vi "Mode Page.vi"(8 "Error in":errorcluster, 11 "INL DNL Test in":refnum<class "INL DNL Test.lvclass">=refnum) -> (0 "Error out":errorcluster, 3 "INL DNL Test out":refnum<class "INL DNL Test.lvclass">)   [LabVIEW 2020, in "INL DNL Test.lvclass"]
doc: "Mode page to select the device mode and enter the device values."
uses:
  INL DNL Test.lvclass
  D:/SDLC/Class/INL DNL Test/Test/Parent/Test.lvclass
  Class/INL DNL Test/Device/Children/Children/ADC/ADC.lvclass
  Class/INL DNL Test/Device/Children/Children/DAC/DAC.lvclass
  Typedef/User event controls.ctl
  Typedef/Queue Operation.ctl
  Class/INL DNL Test/Device/Parent/Device.lvclass
  INL DNL Test.lvclass/INL DNL Test.ctl
  DNL INL Test.lvlib
panel:
  in  "Error Rate (in %)":dbl=25.0 min=0.0 max=100.0
  in  "Voltage (V)":dbl=8.0 min=0.0
  in  "Resolution":dbl=3.0 min=1.0
  in  "DAC":bool caption="Digital to Analog converter"
  in  "ADC":bool caption="Analog to digital converter"
  # "Note:\n1. Choose the mode to calculate INL and DNl result\n2. Enter the parameter values for the calculation"
  # "Choose the mode"
  # "Enter parameters"
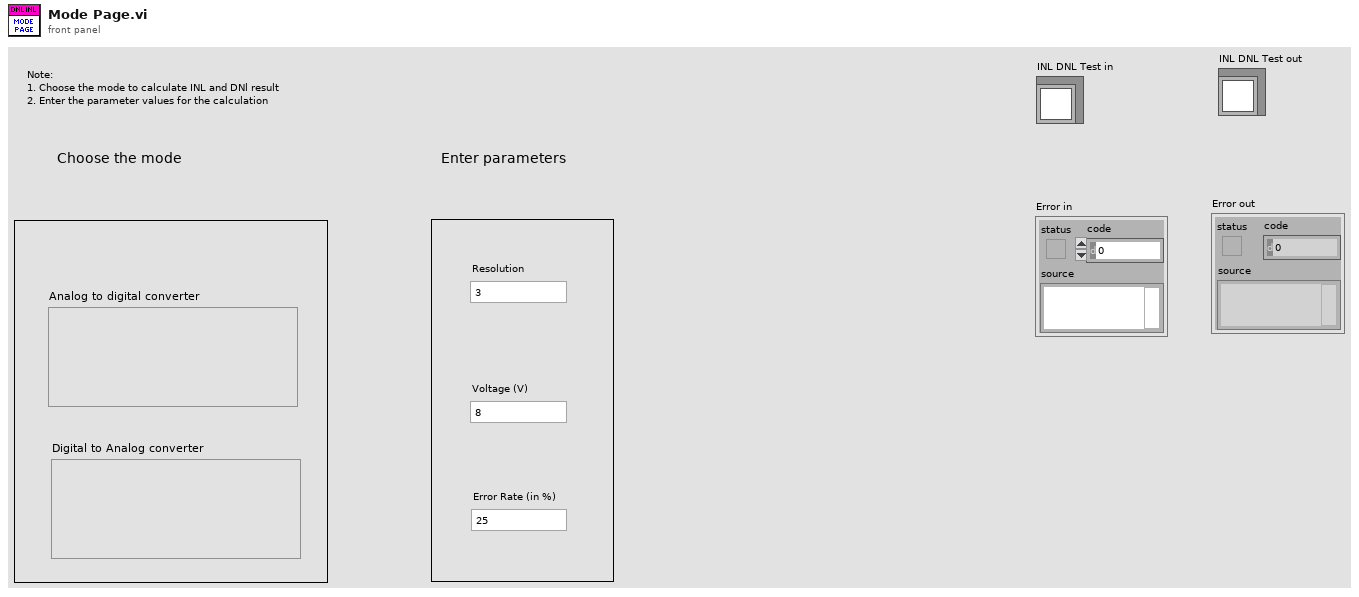
[diagram p1: front panel]
types:
  T1 = typedef "DNL INL Test.lvlib/Queue Operation.ctl" = enum16{"Create Queue", "Enqueue", "Dequeue", "Enstack", "Flush Queue", "Release Queue"}
  T2 = typedef "DNL INL Test.lvlib/User event controls.ctl" = enum16{"Create", "Generate", "Run Test", "Get Ref", "Destroy"}
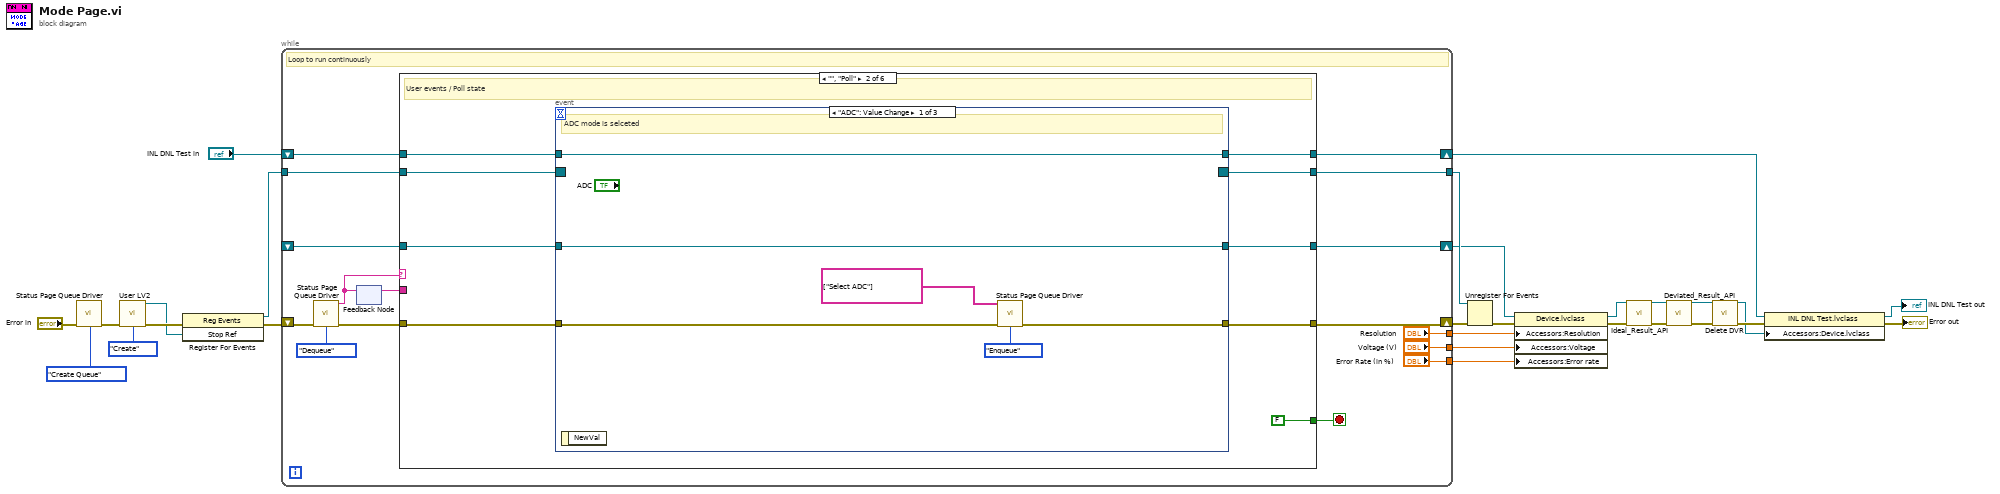
[diagram p0: block diagram]
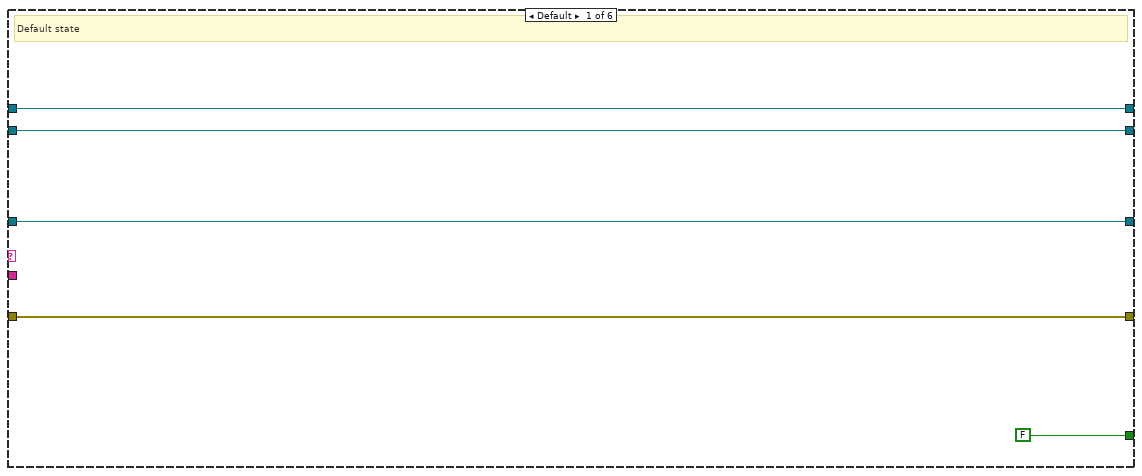
[diagram p2: hidden frame]
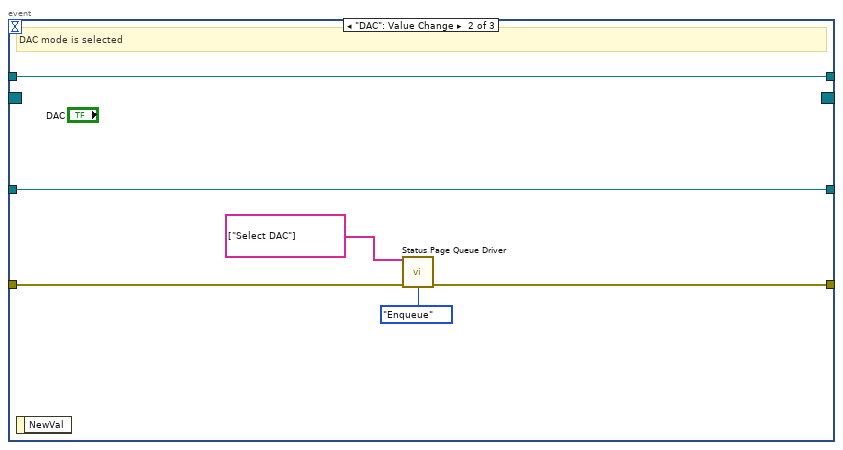
[diagram p3: hidden frame]
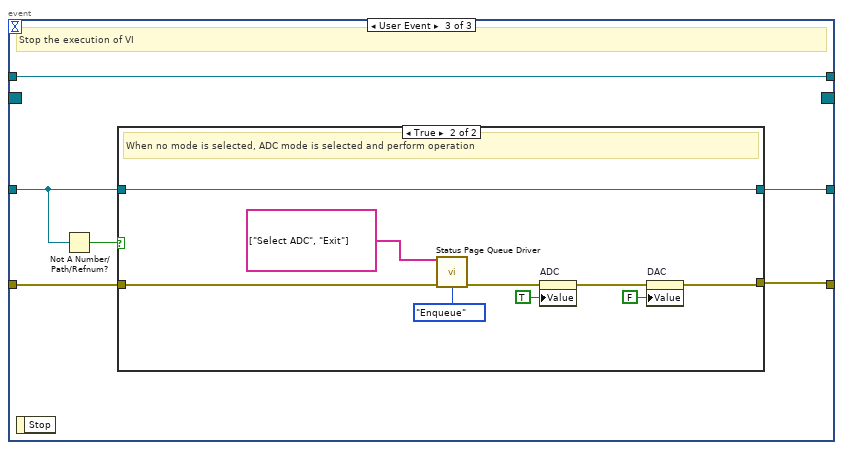
[diagram p4: hidden frame]
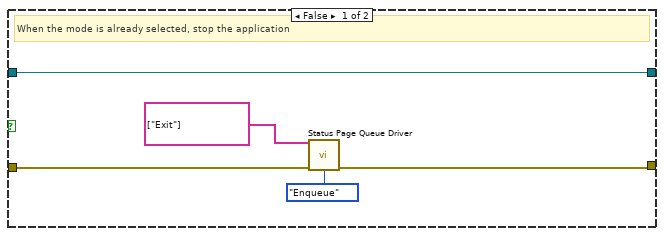
[diagram p5: hidden frame]
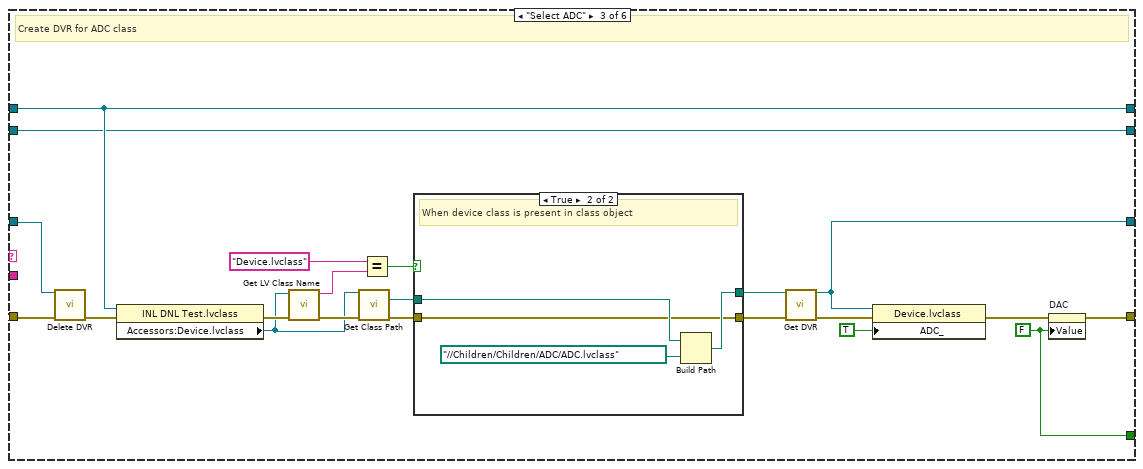
[diagram p6: hidden frame]
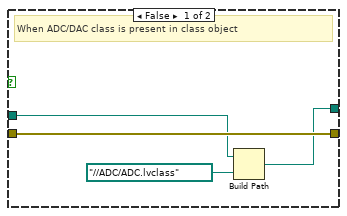
[diagram p7: hidden frame]
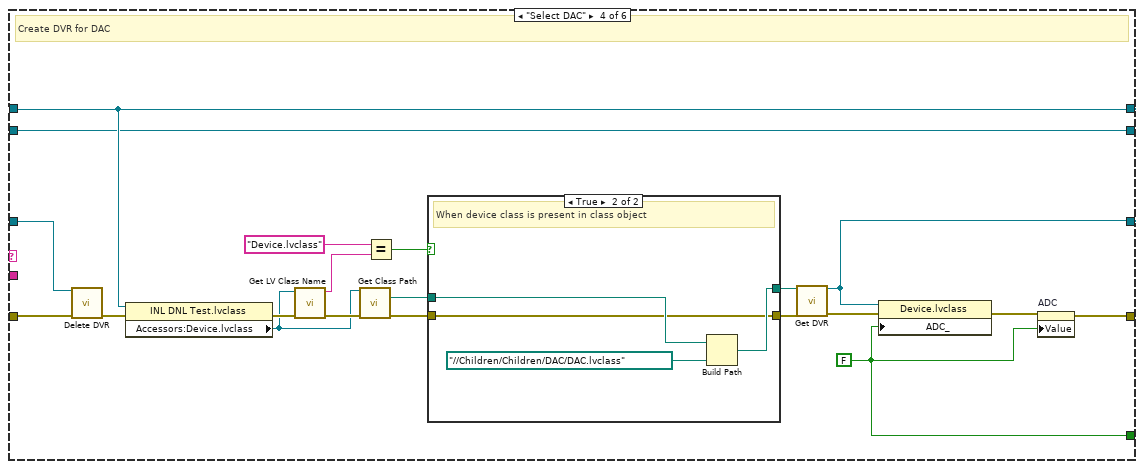
[diagram p8: hidden frame]
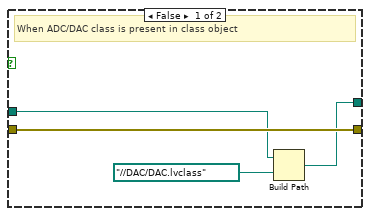
[diagram p9: hidden frame]
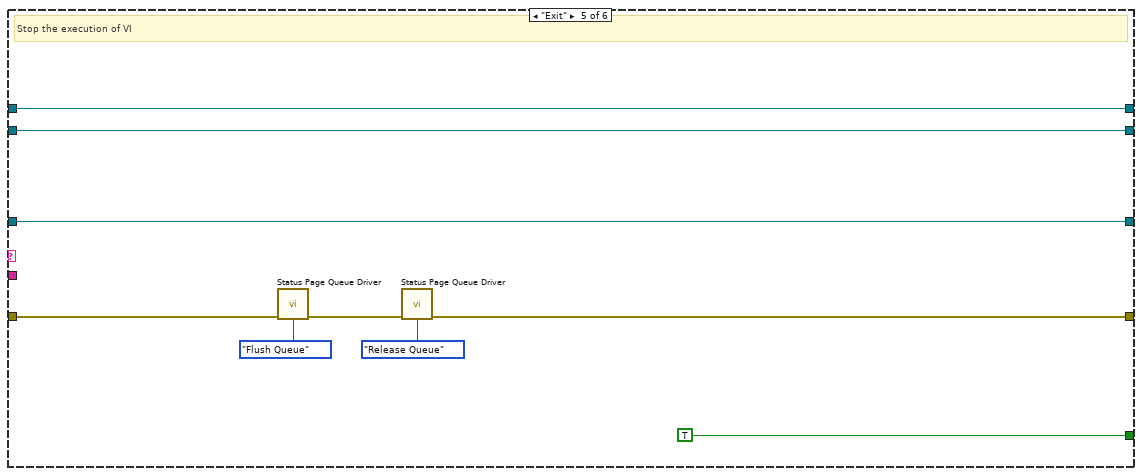
[diagram p10: hidden frame]
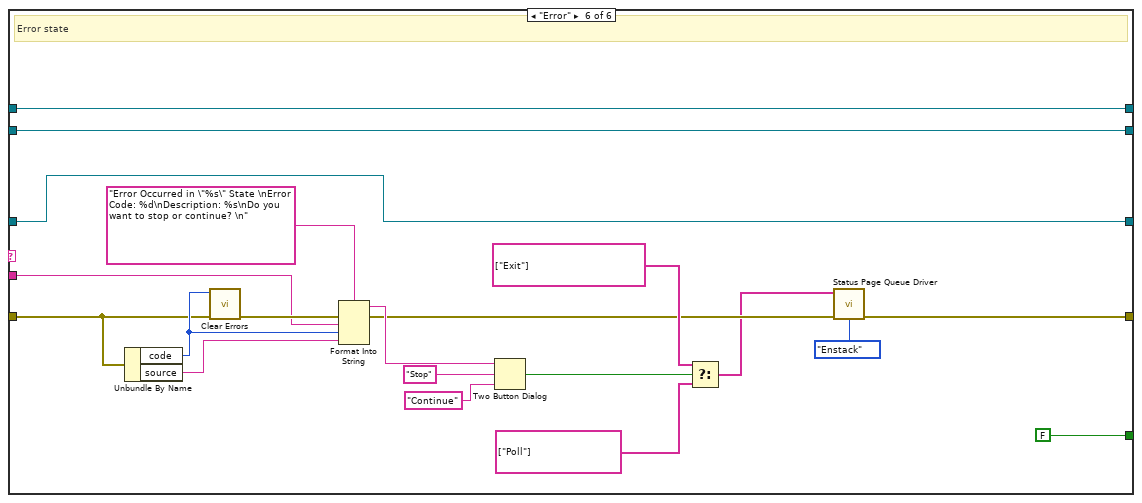
[diagram p11: hidden frame]
diagram:
  n1 = call "Status Page Queue Driver.vi"("Error in"="Error in", "Queue Operation"=Queue_Operation."Create Queue") -> ("Error out"=w5:errorcluster)  [unwired: 12 in, 1 out]
  n2 = call "User LV2.vi"("Error In"=w5, "User event controls"=User_event_controls."Create") -> ("Stop Ref"=w25:refnum<user-event>, "Error Out"=w26:errorcluster)  [unwired: 11 in, 1 out]
  n3 = register-events(error in=w26, w25) -> (reference out=w24:refnum<event-registration>, error out=w23:errorcluster)  [unwired: 1 in]
  n4 = while {
    tunnel: w24 -> [w43]
    shift-right: [w41] -> w14
    shift-left: "INL DNL Test in" -> [w42]
    shift-right: [w40] -> w21
    shift-left: w23 -> [w36]
    tunnel: [w39] -> w19
    shift-right: [w38] -> w18
    shift-left: _ -> [w37]
    tunnel: ["Resolution"] -> w3
    tunnel: ["Error Rate (in %)"] -> w2
    tunnel: ["Voltage (V)"] -> w1
    stop <- w33 stop-if-true
    # "Loop to run continuously"
    n5 = call "Status Page Queue Driver.vi"("Error in"=w36, "Queue Operation"=Queue_Operation."Dequeue") -> ("Dequeue Element"=w29:string, "Error out"=w35:errorcluster)  [unwired: 12 in]
    n6 = feedback-in #1(w29) -> ()
    n7 = feedback #1() -> (w28:string)  [unwired: 1 in]
    n8 = case shown="\"\", \"Poll\"" w29 {
      tunnel: w43 -> [w45 w57 w91 w120 w154 w158]
      tunnel: w35 -> [w46 w56 w96 w125 w151 w165]
      tunnel: w42 -> [w48 w55 w92 w121 w155 w157]
      tunnel: [w48 w54 w92 w121 w155 w157] -> w41
      tunnel: [w46 w53 w93 w122 w149 w160] -> w40
      tunnel: [w45 w52 w91 w120 w154 w158] -> w39
      tunnel: [w47 w51 w94 w123 w153 w159] -> w38
      tunnel: w37 -> [w47 w50 w95 w124 w153 w159]
      tunnel: [FALSE FALSE w90 w119 TRUE FALSE ("ADC_")] -> w33
      tunnel: w28 -> [_ _ _ _ _ w164]
      frame Default {
        # "Default state"
      }
      frame "", "Poll" {
        # "User events / Poll state"
        n9 = event shown="[0] \"ADC\": Value Change" {
          selector: w57 -> [_ _ _]
          dyn-events: [_ _ _] -> w52
          timeout: _ -> [_ _ _]
          tunnel: w56 -> [w61 w67 w75]
          tunnel: w55 -> [w63 w69 w74]
          tunnel: [w63 w69 w74] -> w54
          tunnel: [w60 w64 w73] -> w53
          tunnel: [w62 w68 w72] -> w51
          tunnel: w50 -> [w62 w68 w70]
          event "ADC": Value Change {
            # "ADC mode is selceted"
            n10 = event-data() -> ()  [unwired: 1 in, 1 out]
            n11 = call "Status Page Queue Driver.vi"("States"=string[] ["Select ADC"], "Error in"=w61, "Queue Operation"=Queue_Operation."Enqueue") -> ("Error out"=w60:errorcluster)  [unwired: 11 in, 1 out]
          }
          event "DAC": Value Change {
            # "DAC mode is selected"
            n12 = event-data() -> ()  [unwired: 1 in, 1 out]
            n13 = call "Status Page Queue Driver.vi"("States"=string[] ["Select DAC"], "Error in"=w67, "Queue Operation"=Queue_Operation."Enqueue") -> ("Error out"=w64:errorcluster)  [unwired: 11 in, 1 out]
          }
          event User Event {
            # "Stop the execution of VI"
            n14 = event-data() -> ()  [unwired: 1 in, 1 out]
            n15 = Not A Number/Path/Refnum?(number/path/refnum=w70) -> (NaN/Path/Refnum?=w71:bool)
            n16 = case shown="True" w71 {
              tunnel: w75 -> [w79 w89]
              tunnel: [w78 w82] -> w73
              tunnel: w70 -> [w80 w85]
              tunnel: [w80 w85] -> w72
              frame False {
                # "When the mode is already selected, stop the application"
                n17 = call "Status Page Queue Driver.vi"("States"=string[] ["Exit"], "Error in"=w79, "Queue Operation"=Queue_Operation."Enqueue") -> ("Error out"=w78:errorcluster)  [unwired: 11 in, 1 out]
              }
              frame True {
                # "When no mode is selected, ADC mode is selected and perform operation"
                n18 = call "Status Page Queue Driver.vi"("States"=string[] ["Select ADC", "Exit"], "Error in"=w89, "Queue Operation"=Queue_Operation."Enqueue") -> ("Error out"=w87:errorcluster)  [unwired: 11 in, 1 out]
                n19 = property on="ADC" class="Bool (strict)"(error in=w87, "Value"=TRUE ("ADC")) -> (error out=w84:errorcluster)  [unwired: 1 in, 1 out]
                n20 = property on="DAC" class="Bool (strict)"(error in=w84, "Value"=FALSE ("DAC")) -> (error out=w82:errorcluster)  [unwired: 1 in, 1 out]
              }
            }
          }
        }
      }
      frame "Select ADC" {
        w90 = FALSE ("Digital to Analog converter")
        # "Create DVR for ADC class"
        n21 = call "Delete DVR.vi"("Device DVR"=w95, "Error in"=w96) -> ("Error out"=w108:errorcluster)  [unwired: 12 in, 1 out]
        n22 = property class="INL DNL Test.lvclass"(reference=w92, error in=w108) -> (error out=w104:errorcluster, "Accessors:Device.lvclass"=w102:refnum<class "Device.lvclass">)  [unwired: 1 out]
        n23 = call <vilib>:"Get LV Class Name.vi"("error in (no error)"=w104, "object"=w102) -> ("error out"=w103:errorcluster, "class name"=w101:string)  [unwired: 8 in]
        n24 = call "Get Class Path.vi"("Device in"=w102, "Error in"=w103) -> ("Class Path"=w105:path, "Error out"=w99:errorcluster)  [unwired: 11 in, 1 out]
        n25 = Equal?(x="Device.lvclass", y=w101) -> (x = y?=w97:bool)
        n26 = case shown="True" w97 {
          tunnel: [w111 w118] -> w109
          tunnel: w105 -> [w113 w117]
          tunnel: w99 -> [w114 w115]
          tunnel: [w114 w115] -> w98
          frame False {
            # "When ADC/DAC class is present in class object"
            n27 = Build Path(base path=w113, name or relative path=path "../../ADC/ADC.lvclass") -> (appended path=w111:path)
          }
          frame True {
            # "When device class is present in class object"
            n28 = Build Path(base path=w117, name or relative path=path "../../Children/Children/ADC/ADC.lvclass") -> (appended path=w118:path)
          }
        }
        n29 = call "Get DVR.vi"("Class Path"=w109, "Error in"=w98) -> ("Device DVR"=w94:refnum<data-value>, "Error out"=w110:errorcluster)  [unwired: 12 in]
        n30 = property class="Device.lvclass"(reference=w94, error in=w110, "ADC_"=TRUE) -> (error out=w107:errorcluster)  [unwired: 1 out]
        n31 = property on="DAC" class="Bool (strict)"(error in=w107, "Value"=w90) -> (error out=w93:errorcluster)  [unwired: 1 in, 1 out]
      }
      frame "Select DAC" {
        w119 = FALSE ("ADC_")
        # "Create DVR for DAC"
        n32 = call "Delete DVR.vi"("Device DVR"=w124, "Error in"=w125) -> ("Error out"=w136:errorcluster)  [unwired: 12 in, 1 out]
        n33 = property class="INL DNL Test.lvclass"(reference=w121, error in=w136) -> (error out=w128:errorcluster, "Accessors:Device.lvclass"=w126:refnum<class "Device.lvclass">)  [unwired: 1 out]
        n34 = call <vilib>:"Get LV Class Name.vi"("error in (no error)"=w128, "object"=w126) -> ("error out"=w127:errorcluster, "class name"=w131:string)  [unwired: 8 in]
        n35 = call "Get Class Path.vi"("Device in"=w126, "Error in"=w127) -> ("Class Path"=w134:path, "Error out"=w133:errorcluster)  [unwired: 11 in, 1 out]
        n36 = Equal?(x="Device.lvclass", y=w131) -> (x = y?=w129:bool)
        n37 = case shown="True" w129 {
          tunnel: [w139 w146] -> w137
          tunnel: w134 -> [w141 w145]
          tunnel: w133 -> [w142 w143]
          tunnel: [w142 w143] -> w132
          frame False {
            # "When ADC/DAC class is present in class object"
            n38 = Build Path(base path=w141, name or relative path=path "../../DAC/DAC.lvclass") -> (appended path=w139:path)
          }
          frame True {
            # "When device class is present in class object"
            n39 = Build Path(base path=w145, name or relative path=path "../../Children/Children/DAC/DAC.lvclass") -> (appended path=w146:path)
          }
        }
        n40 = call "Get DVR.vi"("Class Path"=w137, "Error in"=w132) -> ("Device DVR"=w123:refnum<data-value>, "Error out"=w138:errorcluster)  [unwired: 12 in]
        n41 = property class="Device.lvclass"(reference=w123, error in=w138, "ADC_"=w119) -> (error out=w135:errorcluster)  [unwired: 1 out]
        n42 = property on="ADC" class="Bool (strict)"(error in=w135, "Value"=w119) -> (error out=w122:errorcluster)  [unwired: 1 in, 1 out]
      }
      frame "Exit" {
        # "Stop the execution of VI"
        n43 = call "Status Page Queue Driver.vi"("Error in"=w151, "Queue Operation"=Queue_Operation."Flush Queue") -> ("Error out"=w150:errorcluster)  [unwired: 12 in, 1 out]
        n44 = call "Status Page Queue Driver.vi"("Error in"=w150, "Queue Operation"=Queue_Operation."Release Queue") -> ("Error out"=w149:errorcluster)  [unwired: 12 in, 1 out]
      }
      frame "Error" {
        # "Error state"
        n45 = Unbundle By Name(w165) -> ("code"=w173:i32, "source"=w172:string)
        n46 = call <vilib>:"Clear Errors.vi"("error in (no error)"=w165, "specific error code to clear (0: all)"=w173) -> ("error out"=w175:errorcluster)  [unwired: 4 in, 1 out]
        n47 = Format Into String(format string="Error Occurred in \"%s\" State \nError Code: %d\nDescription: %s\nDo you want to stop or continue? \n", error in=w175, w164, w173, w172) -> (resulting string=w171:string, error out=w163:errorcluster)  [unwired: 1 in]
        n48 = Two Button Dialog(message=w171, 1:"Continue" ("F button name (\"Cancel\")"), 2:"Stop" ("T button name (\"OK\")")) -> (T button?=w168:bool)
        n49 = Select(t=string[] ["Exit"] ("States"), s=w168, f=string[] ["Poll"] ("States")) -> (s? t:f=w162:string[])
        n50 = call "Status Page Queue Driver.vi"("States"=w162, "Error in"=w163, "Queue Operation"=Queue_Operation."Enstack") -> ("Error out"=w160:errorcluster)  [unwired: 11 in, 1 out]
      }
    }
  }
  n51 = Unregister For Events(event registration refnum=w19, error in=w21) -> (error out=w20:errorcluster)
  n52 = property class="Device.lvclass"(reference=w18, error in=w20, "Accessors:Resolution"=w3, "Accessors:Voltage"=w1, "Accessors:Error rate"=w2) -> (reference out=w16:refnum<data-value>, error out=w17:errorcluster)
  n53 = call "Ideal_Result_API.vi"("Device DVR"=w16, "Error in"=w17) -> ("Device DVR"=w9:refnum<data-value>, "Error Out"=w10:errorcluster)  [unwired: 12 in]
  n54 = call "Deviated_Result_API.vi"("Device DVR In"=w9, "Error in"=w10) -> ("Device DVR Out"=w7:refnum<data-value>, "Error Out"=w8:errorcluster)  [unwired: 12 in]
  n55 = call "Delete DVR.vi"("Device DVR"=w7, "Error in"=w8) -> ("Device Class Out"=w13:refnum<class "Device.lvclass">, "Error out"=w15:errorcluster)  [unwired: 12 in]
  n56 = property class="INL DNL Test.lvclass"(reference=w14, error in=w15, "Accessors:Device.lvclass"=w13) -> (reference out=→"INL DNL Test out":refnum<class "INL DNL Test.lvclass">, error out=→"Error out":errorcluster)
